vi "LC1_MS_Main.vi"(0 "MS_Network_Settings":T8, 1 "Analog Output":T2[](array[typedef]) {"value" format="%#_15f"}, 2 "Analog Input Indexes":u16[](array[numeric]), 5 "input cluster":T12={"Binary Out Mode"=6, "Binary In Variation"=0, "Analog Out Variation"=4, "Analog Out Mode"=6, "Analog In Variation"=6} {"Binary Out Mode" items=["SBO"=0, "Select"=3, "Operate"=4, "Direct"=5, "Direct No Ack"=6]; "Binary In Variation" items=["Default", "Packed Format", "With Flags"]; "Analog Out Variation" items=["32-bit"=1, "16-bit"=2, "Single-prec"=3, "Double-prec"=4]; "Analog Out Mode" items=["SBO"=0, "Select"=3, "Operate"=4, "Direct"=5, "Direct No Ack"=6]; "Analog In Variation" items=["Default", "32-bit with Flag", "16-bit with Flag", "32-bit without Flag", "16-bit without Flag", "Single-prec with Flag", "Double-prec with Flag"]}, 7 "MS_RESET":bool, 9 "MS_ENABLE":bool, 11 "Poll Enable":T9, 12 "DNP3 Session feedback":T11) -> (4 "MS_SETTINGS_CHANGED":bool, 6 "MS_RESET_IND":bool, 8 "Cluster":T10, 10 "Analog Input":dbl[](array[numeric]), 14 "DNP3 Session":T11, 15 "Digital Input":bool[](array[boolean]))   [LabVIEW 2016, in "DNP3_Master_Station_MGCC.lvlib"]
doc: "-----------------------------------------------------------------------------------------------------------------------\nCopyright <2019> <The University of Tennessee at Knoxville and the University of Tennessee Research Foundation>\nThis software is released under BSD-3 a\nhttps://opensource.org/licenses/BSD-3-Clause \nAdditional license options available at https://utrf.tennessee.edu/industry/sample-agreements/\n-----------------------------------------------------------------------------------------------------------------------"
uses:
  DNP3_Master_Station_MGCC.lvlib
  Tab_Master.ctl
  <vilib>/DNP3/DNP3_Master/Operation Mode.ctl
  <vilib>/DNP3/DNP3_Master/Poll Binary Input Variation.ctl
  <vilib>/DNP3/DNP3_Master/Analog Variation.ctl
  <vilib>/DNP3/DNP3_Master/Poll Analog Input Variation.ctl
  <vilib>/DNP3/DNP3_Master/Response Type.ctl
  <vilib>/DNP3/DNP3_Master/Analog Info.ctl
  <vilib>/DNP3/DNP3_Master/Start Stop.ctl
  <vilib>/Utility/error.llb/Error Cluster From Error Code.vi
  <vilib>/ErrorRing/Error Ring.xnode
  <vilib>/DNP3/DNP3_Master/Send Analog Output Block (Blocking).vi
  <vilib>/DNP3/DNP3_Master/Send CROB (Blocking).vi
  <vilib>/DNP3/DNP3_Master/Send Poll Binary Input By AllPoints (Blocking).vi
  <vilib>/DNP3/DNP3_Master/Read Binary Input.vi
  <vilib>/DNP3/DNP3_Master/Read Analog Input.vi
  <vilib>/DNP3/DNP3_Master/Send Poll Analog Input By StartStop (Blocking).vi
  <vilib>/DNP3/DNP3_Master.lvlib
  <resource>/objmgr/dnp3.rc
panel:
  out "Array":T1[](array[typedef])
  out "stop":i32
  out "Numeric":i32
  out "start":u16
  out "Poll":T1[](array[typedef])
  out "Binary Out Mode":T3=6 items=["SBO"=0, "Select"=3, "Operate"=4, "Direct"=5, "Direct No Ack"=6]
  out "Binary In Variation":T4 items=["Default", "Packed Format", "With Flags"]
  out "Analog Out Variation":T5=4 items=["32-bit"=1, "16-bit"=2, "Single-prec"=3, "Double-prec"=4]
  out "Analog Out Mode":T3 items=["SBO"=0, "Select"=3, "Operate"=4, "Direct"=5, "Direct No Ack"=6]
  out "Analog In Variation":T6 items=["Default", "32-bit with Flag", "16-bit with Flag", "32-bit without Flag", "16-bit without Flag", "Single-prec with Flag", "Double-prec with Flag"]
  out "MS_TX_Status_Binary":T7
  out "MS_TX_Status_Analog":T7
  out "MS_RX_Status_Binary":T7
  out "MS_RX_Status_Analog":T7
  out "MS_Network_Settings_Initial":T8
  in  "En_Tx_Di":bool
  in  "En_Tx_An":bool
  in  "En_Rx_Di":bool
  in  "En_Rx_An":bool
  out "object flags":u8[](array[numeric]) format="%08b"
  in  "Channel Setting":T13
  in  "serial port":u16=1
  in  "baud rate (9600)":u32=9600
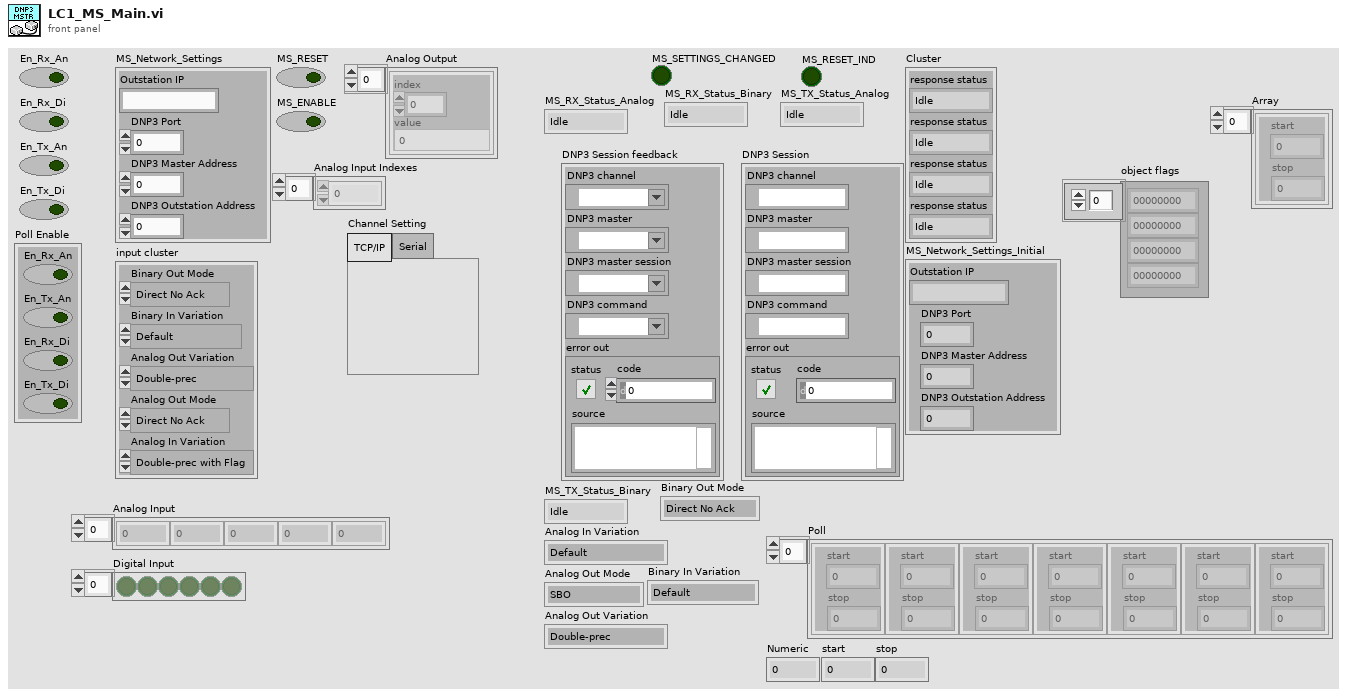
[diagram p1: front panel]
types:
  T1 = typedef "DNP3_Master.lvlib/Start Stop.ctl" = cluster{"start":u16, "stop":u16}
  T2 = typedef "DNP3_Master.lvlib/Analog Info.ctl" = cluster{"index":u16, "value":dbl}
  T3 = typedef "DNP3_Master.lvlib/Operation Mode.ctl" = u8
  T4 = typedef "DNP3_Master.lvlib/Poll Binary Input Variation.ctl" = u8
  T5 = typedef "DNP3_Master.lvlib/Analog Variation.ctl" = u8
  T6 = typedef "DNP3_Master.lvlib/Poll Analog Input Variation.ctl" = u8
  T7 = typedef "DNP3_Master.lvlib/Response Type.ctl" = enum16{"Idle", "Buffering", "Pending", "Success", "Failure", "Mismatch", "Status Code", "IIN", "Timeout", "Cancel"}
  T8 = cluster{"Outstation IP":string, "DNP3 Port":u16, "DNP3 Master Address":u16, "DNP3 Outstation Address":u16}
  T9 = cluster{"En_Rx_An":bool, "En_Tx_An":bool, "En_Rx_Di":bool, "En_Tx_Di":bool}
  T10 = cluster{"response status":T7, "response status":T7, "response status":T7, "response status":T7}
  T11 = cluster{"DNP3 channel":refnum<k21>, "DNP3 master":refnum<k21>, "DNP3 master session":refnum<k21>, "DNP3 command":refnum<k21>, "error out":errorcluster}
  T12 = cluster{"Binary Out Mode":T3, "Binary In Variation":T4, "Analog Out Variation":T5, "Analog Out Mode":T3, "Analog In Variation":T6}
  T13 = typedef "Tab_Master.ctl" = enum32{"TCP/IP", "Serial"}
  T14 = cluster{"Analog RX":T7, "Analog RX":T7, "Analog RX":T7, "Analog RX":T7}
  T15 = cluster{"DNP3 Master Address":u16, "DNP3 Outstation Address":u16}
  T16 = cluster{bool, "Outstation IP":string, "DNP3 Port":u16, "serial port":u16, "baud rate (9600)":u32}
  T17 = typedef "DNP3_Master.lvlib/Crob With Index.ctl" = cluster{"point index":u16, "CROB value":T18}
  T18 = typedef "DNP3_Common.lvlib/crob.ctl" = cluster{"OnTime":u32, "Count":u8, "OffTime":u32, "Control":T19}
  T19 = typedef "DNP3_Common.lvlib/crob_ctrl.ctl" = u8
  T20 = cluster{"MS_RX_Status_Analog":T7, "MS_TX_Status_Analog":T7, "MS_RX_Status_Binary":T7, "MS_TX_Status_Binary":T7}
  T21 = cluster{"DNP3 channel":refnum<k21>, "DNP3 master":refnum<k21>, "DNP3 master session":refnum<k21>, "DNP3 command":refnum<k21>, "error IO":errorcluster}
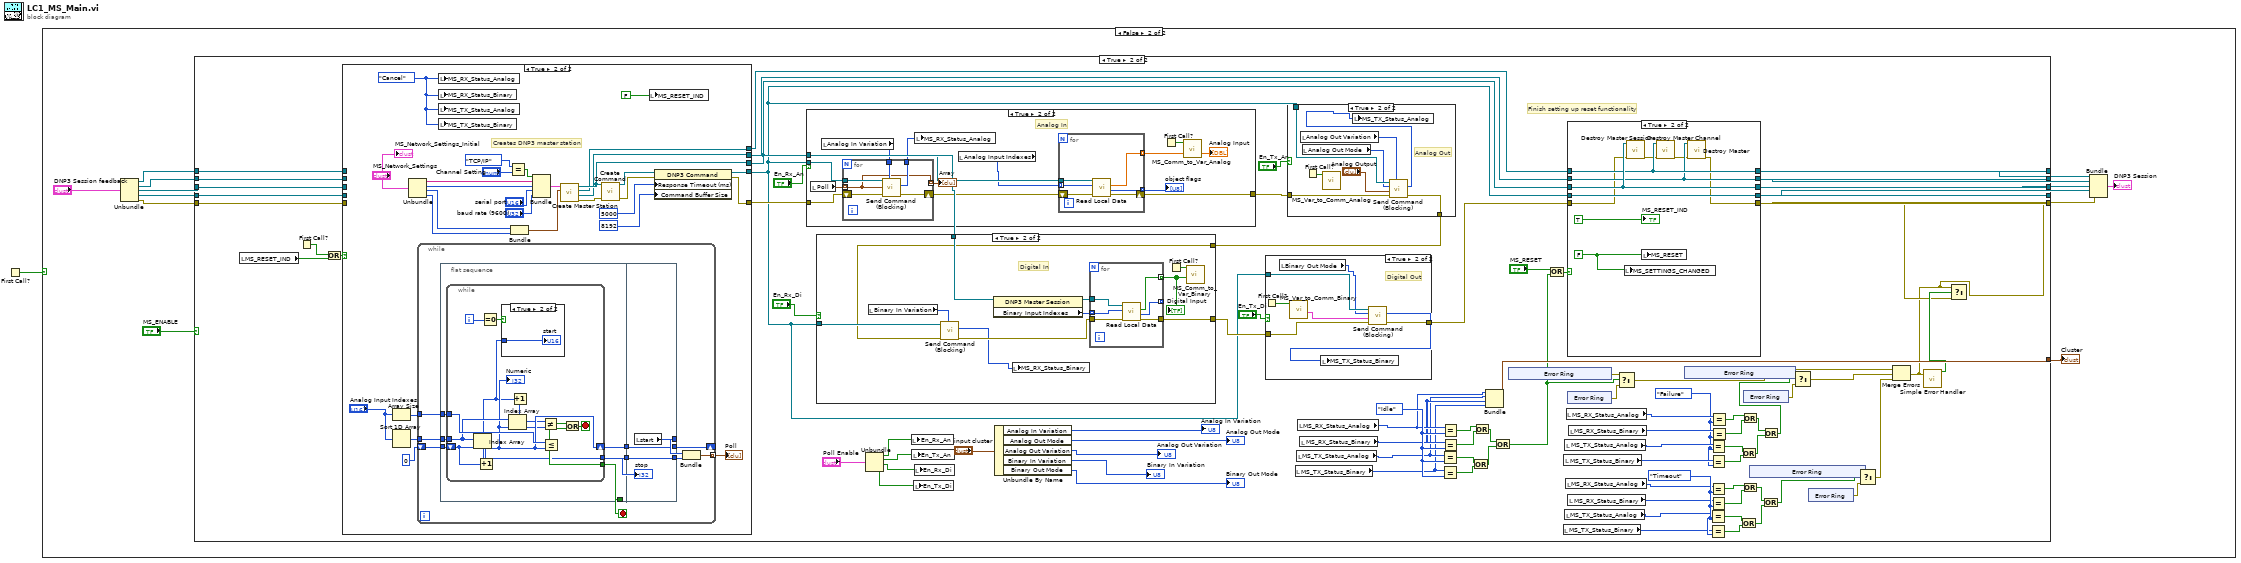
[diagram p0: block diagram]
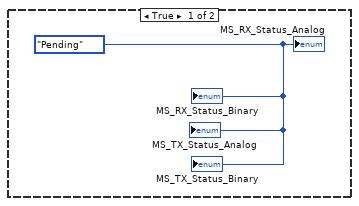
[diagram p2: hidden frame]
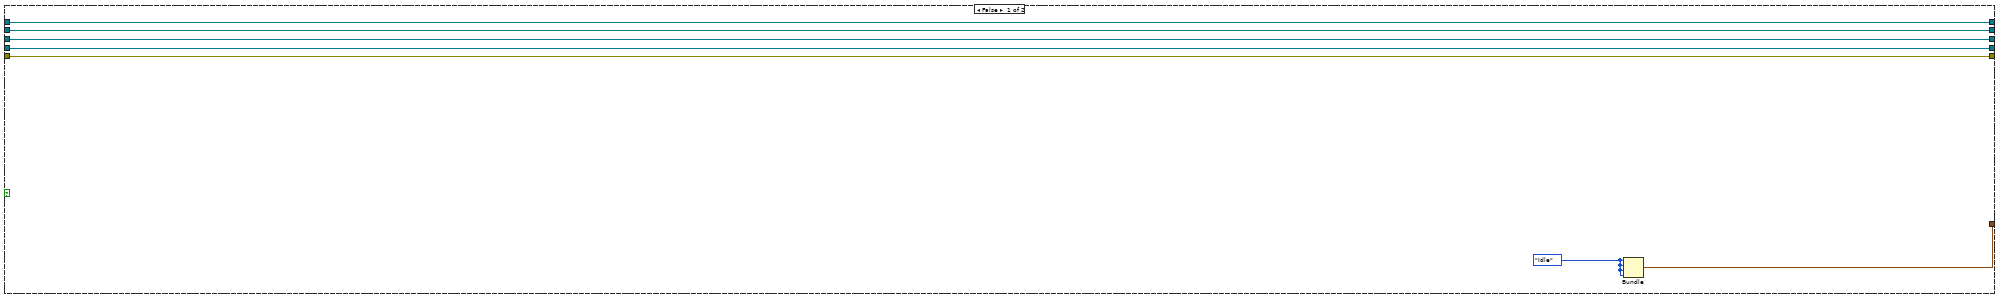
[diagram p3: hidden frame]
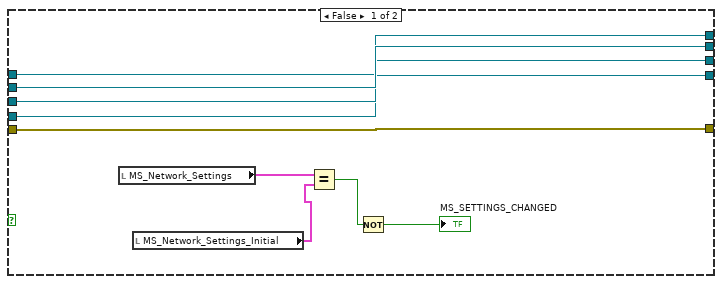
[diagram p9: hidden frame]
diagram:
  n1 = First Call?() -> (First Call?: T/F=w1:bool)
  n2 = case shown="False" w1 {
    frame True {
      w2 = Response_Type."Pending" ("LC1_MS_RX_Status_Binary")
      "MS_RX_Status_Analog" <- w2
      "MS_RX_Status_Binary" <- w2
      "MS_TX_Status_Analog" <- w2
      "MS_TX_Status_Binary" <- w2
    }
    frame False {
      n3 = Unbundle("DNP3 Session feedback") -> ("DNP3 channel"=w16:refnum<k21>, "DNP3 master"=w15:refnum<k21>, "DNP3 master session"=w13:refnum<k21>, "DNP3 command"=w14:refnum<k21>, "error out"=w12:errorcluster)
      n4 = case shown="True" "MS_ENABLE" {
        tunnel: w15 -> [w23 w107]
        tunnel: w13 -> [w22 w106]
        tunnel: w14 -> [w21 w105]
        tunnel: [w23 w103] -> w7
        tunnel: w12 -> [w20 w102]
        tunnel: [w20 w24] -> w4
        tunnel: [w22 w101] -> w6
        tunnel: [w21 w99] -> w5
        tunnel: [w19 w88] -> w8
        tunnel: w16 -> [w19 w87]
        tunnel: [w18 w83] -> w9
        frame False {
          w17 = Response_Type."Idle" ("Analog RX")
          n5 = Bundle("Analog RX"=w17, "Analog RX"=w17, "Analog RX"=w17, "Analog RX"=w17) -> (w18:T14)  [unwired: 1 in]
        }
        frame True {
          w46 = Response_Type."Timeout" ("Analog RX")
          w47 = Response_Type."Failure" ("Analog RX")
          w96 = Response_Type."Idle" ("Analog RX")
          # "Finish setting up reset functionality"
          n6 = local read "MS_RESET_IND"() -> (w69:bool)
          n7 = First Call?() -> (First Call?: T/F=w109:bool)
          n8 = Or(x=w109, y=w69) -> (x .or. y?=w108:bool)
          n9 = case shown="True" w108 {
            tunnel: [w212 w228] -> w110
            tunnel: [w210 w229] -> w79
            tunnel: [w211 w236] -> w100
            tunnel: w107 -> [w213 _]
            tunnel: w106 -> [w211 _]
            tunnel: w105 -> [w210 _]
            tunnel: [w213 w223] -> w104
            tunnel: w102 -> [w212 _]
            tunnel: [w209 w222] -> w89
            tunnel: w87 -> [w209 _]
            frame False {
              n10 = local read "MS_Network_Settings"() -> (w206:T8)
              n11 = local read "MS_Network_Settings_Initial"() -> (w205:T8)
              n12 = Equal?(x=w206, y=w205) -> (x = y?=w207:bool)
              n13 = Not(x=w207) -> (.not. x?=→"MS_SETTINGS_CHANGED":bool)
            }
            frame True {
              w219 = Response_Type."Cancel" ("LC1_MS_RX_Status_Binary")
              # "Creates DNP3 master station"
              n14 = Array Size(array="Analog Input Indexes") -> (size(s)=w216:i32)
              n15 = Sort 1D Array(array="Analog Input Indexes") -> (sorted array=w215:u16[])
              n16 = Unbundle("MS_Network_Settings") -> ("Outstation IP"=w235:string, "DNP3 Port"=w234:u16, "DNP3 Master Address"=w233:u16, "DNP3 Outstation Address"=w232:u16)
              n17 = while {
                tunnel: w215 -> [w251]
                tunnel: w216 -> [w252]
                shift-right: [w250] -> _
                shift-left: 0 -> [w249]
                tunnel: [w248] -> w218 mode=indexing
                stop <- w245 stop-if-true
                n18 = flat-sequence {
                  tunnel: w252 -> [w258]
                  tunnel: w251 -> [w257]
                  tunnel: w249 -> [w255]
                  tunnel: [w256] -> w247
                  tunnel: [w254] -> w245
                  tunnel: [w253] -> w244
                  tunnel: [w274] -> w250
                  tunnel: w247 -> [w274]
                  tunnel: [w273] -> w246
                  tunnel: w244 -> [w272]
                  tunnel: [w272] -> w243
                  frame #0 {
                    n19 = while {
                      tunnel: w258 -> [w270]
                      tunnel: w257 -> [w263]
                      shift-right: [w262] -> w256
                      shift-left: w255 -> [w269]
                      tunnel: [w264] -> w254
                      tunnel: [w259] -> w253
                      i -> [w266]
                      stop <- w268 stop-if-true
                      n20 = Index Array(array=w263, index=w269) -> (element=w259:u16)
                      n21 = Increment(x=w269) -> (x+1=w262:i32)
                      "Numeric" <- w262
                      n22 = Equal To 0?(x=w266) -> (x = 0?=w265:bool)
                      n23 = case shown="True" w265 {
                        tunnel: w259 -> [_ w271]
                        frame False {
                        }
                        frame True {
                          "start" <- w271
                        }
                      }
                      n24 = Index Array(array=w263, index=w262) -> (element=w260:u16)
                      n25 = Increment(x=w259) -> (x+1=w261:u16)
                      n26 = Not Equal?(x=w261, y=w260) -> (x != y?=w267:bool)
                      n27 = Less Or Equal?(x=w270, y=w262) -> (x <= y?=w264:bool)
                      n28 = Or(x=w267, y=w264) -> (x .or. y?=w268:bool)
                    }
                  }
                  frame #1 {
                    n29 = local read "start"() -> (w273:u16)
                    "stop" <- w272
                  }
                }
                n30 = Bundle("start"=w246, w243) -> (w248:cluster{"start":u16, u16})  [unwired: 1 in]
              }
              "Poll" <- w218
              n31 = local write "MS_RX_Status_Analog"(w219) -> ()
              n32 = local write "MS_RX_Status_Binary"(w219) -> ()
              n33 = local write "MS_TX_Status_Analog"(w219) -> ()
              n34 = local write "MS_TX_Status_Binary"(w219) -> ()
              n35 = Equal?(x=Tab_Master."TCP/IP" ("Channel Setting"), y="Channel Setting") -> (x = y?=w238:bool)
              n36 = Bundle("DNP3 Master Address"=w233, "DNP3 Outstation Address"=w232) -> (w230:T15)  [unwired: 1 in]
              n37 = Bundle(w238, "Outstation IP"=w235, "DNP3 Port"=w234, "serial port"="serial port", "baud rate (9600)"="baud rate (9600)") -> (w231:T16)  [unwired: 1 in]
              n38 = call "Create Master Station.vi"("Session Cluster"=w230, "Channel Cluster"=w231) -> ("error out"=w239:errorcluster, "DNP3 master"=w223:refnum<k21>, "DNP3 channel"=w222:refnum<k21>, "DNP3 master session"=w236:refnum<k21>)  [unwired: 3 in]
              n39 = call <vilib>:"Create Command.vi"("error in (no error)"=w239, "DNP3 master session"=w236) -> ("error out"=w226:errorcluster, "DNP3 command"=w227:refnum<k21>)  [unwired: 8 in]
              n40 = local write "MS_RESET_IND"(FALSE ("MS_Comm_Reset_Ind")) -> ()
              n41 = property class="DNP3 Command"(reference=w227, error in=w226, "Response Timeout (ms)"=u32 5000 ("Misc:Response Timeout (ms)"), "Command Buffer Size"=u32 8192 ("Misc:Command Buffer Size")) -> (reference out=w229:refnum<k21>, error out=w228:errorcluster)
              "MS_Network_Settings_Initial" <- "MS_Network_Settings"
            }
          }
          n42 = case shown="True" "En_Rx_An" {
            tunnel: w110 -> [w164 w177]
            tunnel: w100 -> [_ w169]
            tunnel: w79 -> [_ w176]
            tunnel: [w164 w174] -> w82
            frame False {
            }
            frame True {
              # "Analog In"
              n43 = local read "Poll"() -> (w167:T1[])
              n44 = local read "Analog In Variation"() -> (w170:T6)
              n45 = for {
                tunnel: w176 -> [w182]
                tunnel: [w181] -> w171
                tunnel: w170 -> [w180]
                shift-right: [w179] -> w168
                shift-left: w177 -> [w183]
                tunnel: w167 -> [w178] mode=indexing
                tunnel: [w178] -> w165 mode=indexing
                n46 = call-poly <vilib>:"Send Command (Blocking).vi"("variation (Default)"=w180, "error in (no error)"=w183, "range"=w178, "DNP3 command in"=w182) -> ("error out"=w179:errorcluster, "response status"=w181:T7)  [unwired: 5 in, 1 out]
              }
              "Array" <- w165
              n47 = local write "MS_RX_Status_Analog"(w171) -> ()
              n48 = local read "Analog Input Indexes"() -> (w166:u16[])
              n49 = for {
                tunnel: [w187] -> w172 mode=indexing
                tunnel: [w186] -> w175 mode=indexing
                tunnel: w169 -> [w185]
                tunnel: w166 -> [w184] mode=indexing
                shift-right: [w188] -> w174
                shift-left: w168 -> [w189]
                n50 = call-poly <vilib>:"Read Local Data.vi"("error in (no error)"=w189, "point index"=w184, "DNP3 master session in"=w185) -> ("error out"=w188:errorcluster, "object flags"=w186:u8, "value"=w187:dbl)  [unwired: 5 in, 1 out]
              }
              "object flags" <- w175
              "Analog Input" <- w172
              n51 = First Call?() -> (First Call?: T/F=w173:bool)
              n52 = call "MS_Comm_to_Var_Analog.vi"("Array"=w172, "Boolean"=w173) -> ()  [unwired: 10 in]
            }
          }
          n53 = Unbundle("Poll Enable") -> ("En_Rx_An"=w74:bool, "En_Tx_An"=w73:bool, "En_Rx_Di"=w72:bool, "En_Tx_Di"=w71:bool)
          n54 = local write "En_Rx_An"(w74) -> ()
          n55 = local write "En_Tx_An"(w73) -> ()
          n56 = local write "En_Tx_Di"(w71) -> ()
          n57 = local write "En_Rx_Di"(w72) -> ()
          n58 = Unbundle By Name("input cluster") -> ("Analog In Variation"=→"Analog In Variation":T6, "Analog Out Mode"=→"Analog Out Mode":T3, "Analog Out Variation"=→"Analog Out Variation":T5, "Binary In Variation"=→"Binary In Variation":T4, "Binary Out Mode"=→"Binary Out Mode":T3)
          n59 = case shown="True" "En_Tx_An" {
            tunnel: w79 -> [_ w163]
            tunnel: w82 -> [w155 w162]
            tunnel: [w155 w161] -> w81
            frame False {
            }
            frame True {
              # "Analog Out"
              n60 = local read "Analog Out Variation"() -> (w157:T5)
              n61 = local read "Analog Out Mode"() -> (w158:T3)
              n62 = First Call?() -> (First Call?: T/F=w160:bool)
              n63 = call "MS_Var_to_Comm_Analog.vi"("Boolean"=w160) -> ()  [unwired: 11 in]
              n64 = call-poly <vilib>:"Send Command (Blocking).vi"("variation"=w157, "error in (no error)"=w162, "values"="Analog Output", "mode"=w158, "DNP3 command in"=w163) -> ("error out"=w161:errorcluster, "response status"=w159:T7)  [unwired: 4 in, 1 out]
              n65 = local write "MS_TX_Status_Analog"(w159) -> ()
            }
          }
          n66 = case shown="True" "En_Rx_Di" {
            tunnel: w100 -> [_ w148]
            tunnel: w79 -> [_ w147]
            tunnel: w81 -> [w137 w146]
            tunnel: [w137 w145] -> w80
            frame False {
            }
            frame True {
              # "Digital In"
              n67 = local read "Binary In Variation"() -> (w138:T4)
              n68 = call-poly <vilib>:"Send Command (Blocking).vi"("variation (Default)"=w138, "error in (no error)"=w146, "DNP3 command in"=w147) -> ("error out"=w142:errorcluster, "response status"=w139:T7)  [unwired: 6 in, 1 out]
              n69 = property class="DNP3 Master Session"(reference=w148) -> (reference out=w144:refnum<k21>, "Binary Input Indexes"=w143:u16[])  [unwired: 1 in, 1 out]
              n70 = local write "MS_RX_Status_Binary"(w139) -> ()
              n71 = for {
                tunnel: [w154] -> w145
                tunnel: [w153] -> _ mode=indexing
                tunnel: [w152] -> w141 mode=indexing
                tunnel: w144 -> [w151]
                tunnel: w143 -> [w150] mode=indexing
                tunnel: w142 -> [w149]
                n72 = call-poly <vilib>:"Read Local Data.vi"("error in (no error)"=w149, "point index"=w150, "DNP3 master session in"=w151) -> ("error out"=w154:errorcluster, "object flags"=w153:u8, "value"=w152:bool)  [unwired: 5 in, 1 out]
              }
              "Digital Input" <- w141
              n73 = First Call?() -> (First Call?: T/F=w140:bool)
              n74 = call "MS_Comm_to_Var_Binary.vi"("Input Data"=w141, "Boolean"=w140) -> ()  [unwired: 10 in]
            }
          }
          n75 = case shown="True" "En_Tx_Di" {
            tunnel: [w129 w136] -> w98
            tunnel: w80 -> [w129 w135]
            tunnel: w79 -> [_ w132]
            frame False {
            }
            frame True {
              # "Digital Out"
              n76 = First Call?() -> (First Call?: T/F=w133:bool)
              n77 = local read "Binary Out Mode"() -> (w130:T3)
              n78 = call "MS_Var_to_Comm_Binary.vi"("Boolean"=w133) -> ("Array"=w134:T17[])  [unwired: 10 in]
              n79 = call-poly <vilib>:"Send Command (Blocking).vi"("error in (no error)"=w135, "CROB values"=w134, "mode"=w130, "DNP3 command in"=w132) -> ("error out"=w136:errorcluster, "response status"=w131:T7)  [unwired: 5 in, 1 out]
              n80 = local write "MS_TX_Status_Binary"(w131) -> ()
            }
          }
          n81 = local read "MS_TX_Status_Binary"() -> (w64:T7)
          n82 = local read "MS_TX_Status_Analog"() -> (w65:T7)
          n83 = local read "MS_RX_Status_Analog"() -> (w67:T7)
          n84 = local read "MS_RX_Status_Binary"() -> (w66:T7)
          n85 = Equal?(x=w65, y=w96) -> (x = y?=w91:bool)
          n86 = Equal?(x=w64, y=w96) -> (x = y?=w92:bool)
          n87 = Equal?(x=w67, y=w96) -> (x = y?=w93:bool)
          n88 = Equal?(x=w66, y=w96) -> (x = y?=w90:bool)
          n89 = Or(x=w91, y=w92) -> (x .or. y?=w94:bool)
          n90 = Or(x=w93, y=w90) -> (x .or. y?=w95:bool)
          n91 = Bundle("MS_RX_Status_Analog"=w67, "MS_TX_Status_Analog"=w65, "MS_RX_Status_Binary"=w66, "MS_TX_Status_Binary"=w64) -> (w83:T20)  [unwired: 1 in]
          n92 = Or(x=w95, y=w94) -> (x .or. y?=w52:bool)
          n93 = xnode "Error Ring"() -> ("error out"=w53:errorcluster)
          n94 = Or(x="MS_RESET", y=w52) -> (x .or. y?=w97:bool)
          n95 = local read "MS_TX_Status_Binary"() -> (w45:T7)
          n96 = local read "MS_TX_Status_Binary"() -> (w48:T7)
          n97 = local read "MS_TX_Status_Analog"() -> (w38:T7)
          n98 = local read "MS_TX_Status_Analog"() -> (w60:T7)
          n99 = local read "MS_RX_Status_Analog"() -> (w43:T7)
          n100 = local read "MS_RX_Status_Analog"() -> (w50:T7)
          n101 = case shown="True" w97 {
            tunnel: w104 -> [w194 w200]
            tunnel: [w194 w200] -> w103
            tunnel: w98 -> [w193 w199]
            tunnel: [w193 w196] -> w25
            tunnel: [w192 w202] -> w101
            tunnel: w100 -> [w192 w202]
            tunnel: [w191 w204] -> w99
            tunnel: w79 -> [w191 w204]
            tunnel: w89 -> [w190 w201]
            tunnel: [w190 w201] -> w88
            frame False {
            }
            frame True {
              w195 = FALSE ("MS_Comm_Reset")
              n102 = local write "MS_SETTINGS_CHANGED"(w195) -> ()
              n103 = call <vilib>:"Destroy Master Session.vi"("error in (no error)"=w199, "DNP3 master session in"=w202) -> ("error out"=w198:errorcluster)  [unwired: 8 in, 1 out]
              n104 = local write "MS_RESET"(w195) -> ()
              n105 = call <vilib>:"Destroy Master Channel.vi"("error in (no error)"=w198, "DNP3 channel in"=w201) -> ("error out"=w197:errorcluster)  [unwired: 8 in, 1 out]
              n106 = call <vilib>:"Destroy Master.vi"("error in (no error)"=w197, "DNP3 master"=w200) -> ("error out"=w196:errorcluster)  [unwired: 9 in]
              "MS_RESET_IND" <- TRUE ("MS_Comm_Reset_Succesful")
            }
          }
          n107 = xnode "Error Ring"() -> ("error out"=w54:errorcluster)
          n108 = local read "MS_RX_Status_Binary"() -> (w44:T7)
          n109 = local read "MS_RX_Status_Binary"() -> (w49:T7)
          n110 = Select(t=w53, s=w52, f=w54) -> (s? t:f=w29:errorcluster)
          n111 = xnode "Error Ring"() -> ("error out"=w35:errorcluster)
          n112 = Equal?(x=w38, y=w46) -> (x = y?=w40:bool)
          n113 = Equal?(x=w45, y=w46) -> (x = y?=w41:bool)
          n114 = Equal?(x=w60, y=w47) -> (x = y?=w58:bool)
          n115 = Equal?(x=w48, y=w47) -> (x = y?=w57:bool)
          n116 = Equal?(x=w43, y=w46) -> (x = y?=w42:bool)
          n117 = Equal?(x=w44, y=w46) -> (x = y?=w39:bool)
          n118 = Equal?(x=w50, y=w47) -> (x = y?=w51:bool)
          n119 = Equal?(x=w49, y=w47) -> (x = y?=w59:bool)
          n120 = Or(x=w40, y=w41) -> (x .or. y?=w36:bool)
          n121 = Or(x=w58, y=w57) -> (x .or. y?=w56:bool)
          n122 = Or(x=w42, y=w39) -> (x .or. y?=w37:bool)
          n123 = Or(x=w51, y=w59) -> (x .or. y?=w55:bool)
          n124 = xnode "Error Ring"() -> ("error out"=w34:errorcluster)
          n125 = xnode "Error Ring"() -> ("error out"=w32:errorcluster)
          n126 = Or(x=w37, y=w36) -> (x .or. y?=w30:bool)
          n127 = Or(x=w55, y=w56) -> (x .or. y?=w31:bool)
          n128 = Select(t=w35, s=w31, f=w34) -> (s? t:f=w28:errorcluster)
          n129 = xnode "Error Ring"() -> ("error out"=w33:errorcluster)
          n130 = Select(t=w32, s=w30, f=w33) -> (s? t:f=w27:errorcluster)
          n131 = Merge Errors(w29, w28, w27) -> (w24:errorcluster)
          n132 = call <vilib>:"Simple Error Handler.vi"("error in (no error)"=w24) -> ("error?"=w26:bool)  [unwired: 4 in, 4 out]
          n133 = Select(t=w24, s=w26, f=w25) -> ()  [unwired: 1 out]
        }
      }
      "Cluster" <- w9
      n134 = Bundle("DNP3 channel"=w8, "DNP3 master"=w7, "DNP3 master session"=w6, "DNP3 command"=w5, "error IO"=w4) -> (→"DNP3 Session":T21)  [unwired: 1 in]
    }
  }
